vi "Get Plugin.vi"(10 "index":i32, 11 "Framework in":refnum<class "Framework.lvclass">) -> (2 "Plugin":refnum<class "Plugin.lvclass">, 3 "Framework out":refnum<class "Framework.lvclass">)   [LabVIEW 2017, in "Data Sharing Framework Core.lvlib" / "Data Sharing Framework Engine.lvlib" / "Framework.lvclass"]
uses:
  Framework.lvclass
  Plugin/Plugin.lvclass
  Framework.lvclass/Framework.ctl
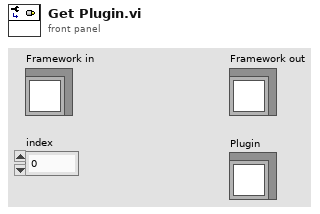
[diagram p1: front panel]
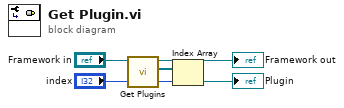
[diagram p0: block diagram]
diagram:
  n1 = call "Get Plugins.vi"("Framework in"="Framework in") -> ("Plugins"=w3:refnum<class "Plugin.lvclass">[], "Framework out"=→"Framework out":refnum<class "Framework.lvclass">)  [unwired: 9 in]
  n2 = Index Array(array=w3, index="index") -> (element=→"Plugin":refnum<class "Plugin.lvclass">)
